vi "习题3.5.vi"() -> ()   [LabVIEW 2018]
panel:
  out "exp(x)":dbl
  out "exp(x)":dbl
  in  "x":dbl
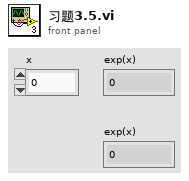
[diagram p1: front panel]
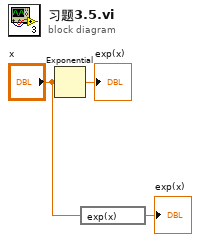
[diagram p0: block diagram]
diagram:
  n1 = Exponential(1:"x") -> (0:→"exp(x)":dbl)
  n2 = expression code="exp(x)"("x") -> (→"exp(x)":dbl)
